vi "remove-set-fromstring.vi"(10 "error in (no error)":errorcluster, 11 "String":string) -> (2 "error out":errorcluster, 3 "result string":string)   [LabVIEW 2020, in "Highland T564 DDG.lvclass"]
uses:
  Highland T564 DDG.lvclass
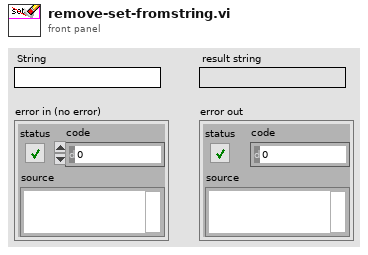
[diagram p1: front panel]
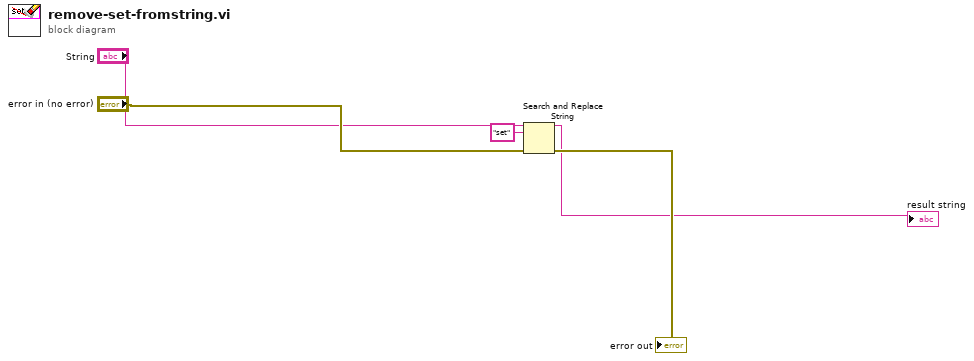
[diagram p0: block diagram]
diagram:
  n1 = Search and Replace String(input string="String", search string="set", error in="error in (no error)") -> (result string=→"result string":string, error out=→"error out":errorcluster)  [unwired: 5 in, 2 out]
